vi "Write Normalized Waveforms to FGEN.vi"(0 "FGEN Resource In":refnum<k15>, 1 "Waveform Names":string[](array[string]), 2 "Resampled Waveforms":waveform(dbl)[](array[waveform]), 3 "error in (no error)":errorcluster) -> (7 "FGEN Resource Out":refnum<k15>, 10 "error out":errorcluster)   [LabVIEW 2025]
uses:
  <instrlib>/niFgen/niFgen.llb/niFgen Write Named Waveform (WDT).vi
  <vilib>/Waveform/WDTOps.llb/WDT Append Waveforms DBL.vi
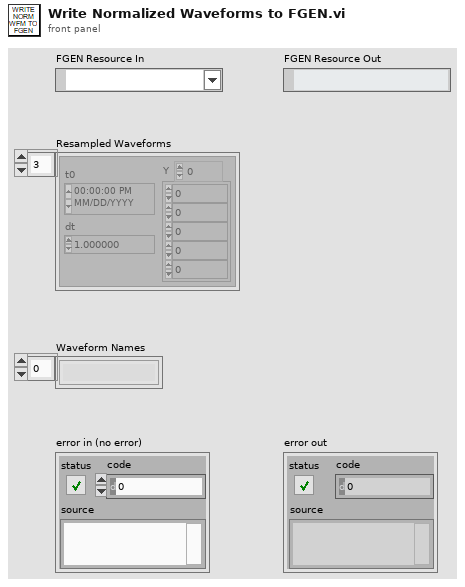
[diagram p1: front panel]
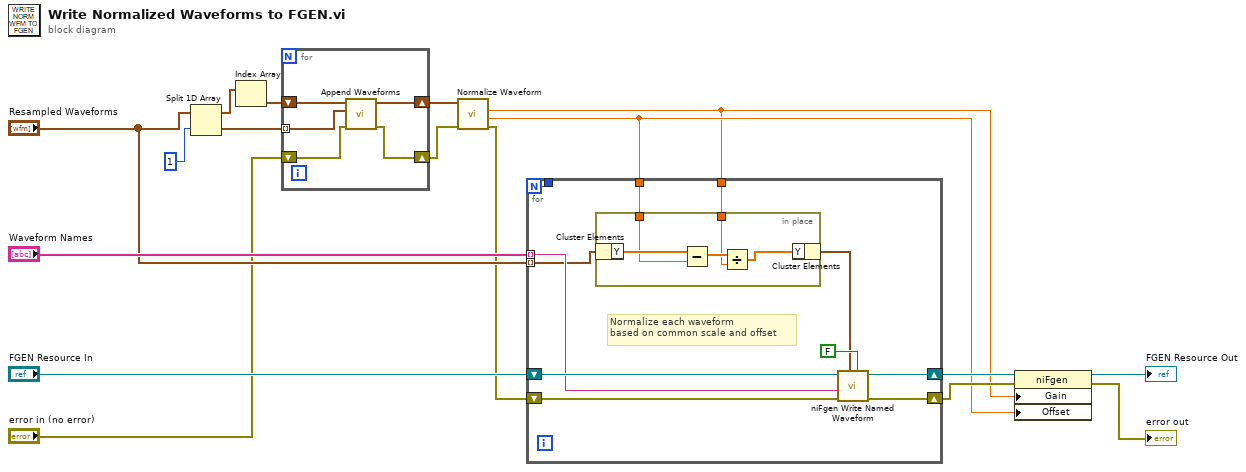
[diagram p0: block diagram]
diagram:
  n1 = Split 1D Array(array="Resampled Waveforms", index=1) -> (first subarray=w15:waveform(dbl)[], second subarray=w17:waveform(dbl)[])
  n2 = Index Array(array=w15) -> (element=w14:waveform(dbl))  [unwired: 1 in]
  n3 = for {
    tunnel: w17 -> [w21] mode=indexing
    shift-right: [w20] -> w13
    shift-left: w14 -> [w22]
    shift-right: [w18] -> w4
    shift-left: "error in (no error)" -> [w19]
    n4 = call-poly <vilib>:"Append Waveforms.vi"("error in (no error)"=w19, "waveform B"=w21, "waveform A"=w22) -> ("error out"=w18:errorcluster, "waveform out"=w20:waveform(dbl))  [unwired: 7 in]
  }
  n5 = call <vilib>:"Normalize Waveform.vi"("error in (no error)"=w4, "waveform in"=w13) -> ("error out"=w3:errorcluster, "offset"=w2:dbl, "scale"=w1:dbl)  [unwired: 6 in, 1 out]
  n6 = for {
    N -> [w27]
    shift-right: [w33] -> w7
    shift-left: w3 -> [w32]
    tunnel: "Resampled Waveforms" -> [w26] mode=indexing
    tunnel: "Waveform Names" -> [w30] mode=indexing
    shift-right: [w28] -> w9
    shift-left: "FGEN Resource In" -> [w31]
    tunnel: [w27] -> _
    tunnel: w2 -> [w24]
    tunnel: w1 -> [w23]
    # "Normalize each waveform\nbased on common scale and offset"
    n7 = in-place {
      in-place-border: w24 -> [w37]
      in-place-border: w23 -> [w35]
      n8 = in-place-cluster #1(w26) -> ("Y"=w38:dbl[])
      n9 = Subtract(x=w38, y=w37) -> (x-y=w36:dbl[])
      n10 = Divide(x=w36, y=w35) -> (x/y=w34:dbl[])
      n11 = in-place-cluster #1("Y"=w34) -> (w25:waveform(dbl))
    }
    n12 = call-poly <instrlib>:"niFgen Write Named Waveform.vi"("Use Waveform dT for Sample Rate"=FALSE, "Waveform"=w25, "error in (no error)"=w32, "Waveform Name"=w30, "Instrument Handle"=w31) -> ("error out"=w33:errorcluster, "Instrument Handle Out"=w28:refnum<k15>)  [unwired: 4 in, 1 out]
  }
  n13 = property class="niFgen"(reference=w9, error in=w7, "Gain"=w1, "Offset"=w2) -> (reference out=→"FGEN Resource Out":refnum<k15>, error out=→"error out":errorcluster)
